vi "Pfeiffer-RVC300.set flow.vi"(0 "i ref in":refnum<vi>, 1 "flow":dbl, 3 "ms timeout (10000)":i32=10000, 5 "error in (no error)":errorcluster) -> (14 "i ref out":refnum<vi>, 17 "timed out":bool, 19 "error out":errorcluster)   [LabVIEW 2014, in "Pfeiffer-RVC300.lvlib"]
doc: "Sets the flow for flow regulation.\n\nLicense Agreement for this software:\n\nCopyright (C)\nMax-Planck-Institut für Kernphysik\nSaupfercheckweg 1\n69117 Heidelberg\nGermany\n\nContact: christopher.borgmann@mpi-hd.mpg.de\n\nThis program is free software: you can redistribute it and/or modify \nit under the terms of the GNU General Public License as published by\nthe Free Software Foundation, either version 3 of the License, or\n(at your option) any later version.\n\nThis program is distributed in the hope that it will be useful,\nbut WITHOUT ANY WARRANTY; without even the implied warranty of\nMERCHANTABILITY or FITNESS FOR A PARTICULAR PURPOSE. See the\nGNU General Public License for more details.\n\nYou should have received a copy of the GNU General Public License\nalong with this program. If not, see <http://www.gnu.org/licenses/>.\n\nMax-Planck-Institut für Kernphysik\nSaupfercheckweg 1, 69117 Heidelberg, Germany\nFor all questions and ideas contact: christopher.borgmann@mpi-hd.mpg.de\nLast update: 08.07.2010"
uses:
  Pfeiffer-RVC300.lvlib
  CSCore/CSApplicationBaseClasses/DeviceBase/DeviceBase.lvlib
  CSlibraries-extern/DimLVEvent/LVDimInterface/LVDimInterface.lvlib
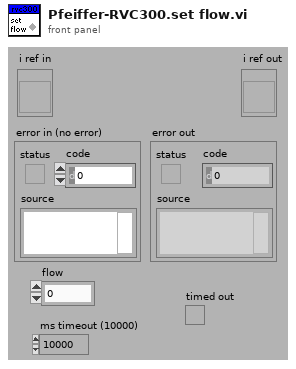
[diagram p1: front panel]
types:
  T1 = typedef "Pfeiffer-RVC300.lvlib/Pfeiffer-RVC300.i attribute.ctl" = cluster{"interfaceInitialized":bool, "VISAResource":refnum<visa-resource-name>, "WaitingTime":u32, "nomValues":T2, "actValues":T2}
  T2 = typedef "Pfeiffer-RVC300.lvlib/Pfeiffer-RVC300.parameters.ctl" = cluster{"regulationMode":T3, "valveType":string, "sensorType":string, "valveState":string, "flow":dbl, "pressure":dbl, "serviceIDs":cluster{"regulationModeID":i32, "valveTypeID":i32, "sensorTypeID":i32, "valveStateID":i32, "flowID":i32, "pressureID":i32}}
  T3 = typedef "Pfeiffer-RVC300.lvlib/Pfeiffer-RVC300.regulation mode.ctl" = enum16{"unknown", "Pressure", "Flow", "Wait"}
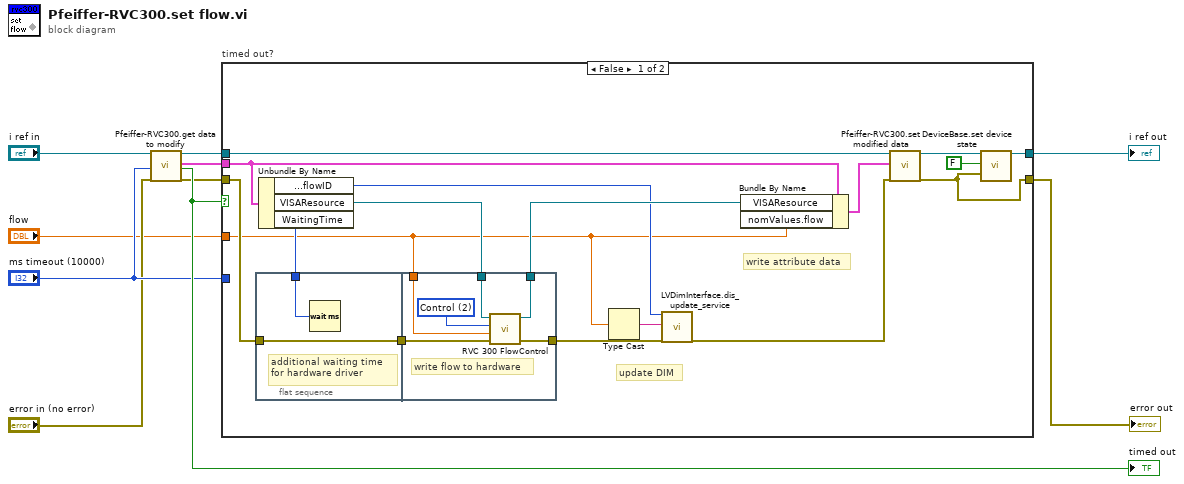
[diagram p0: block diagram]
diagram:
  n1 = call "Pfeiffer-RVC300.get data to modify.vi"("i ref in"="i ref in", "ms timeout (10000)"="ms timeout (10000)", "error in (no error)"="error in (no error)") -> ("i ref out"=w4:refnum<vi>, "i attribute"=w2:T1, "timed out"=w7:bool, "error out"=w3:errorcluster)  [unwired: 13 in]
  "timed out" <- w7
  n2 = case "timed out?" shown="False" w7 {
    tunnel: [w24 w37] -> w9
    tunnel: w4 -> [w27 w37]
    tunnel: [w22 w36] -> w8
    tunnel: w3 -> [w21 w36]
    tunnel: w2 -> [w19 _]
    tunnel: "ms timeout (10000)" -> [_ _]
    tunnel: "flow" -> [w11 _]
    frame False {
      # "write attribute data"
      # "update DIM"
      n3 = flat-sequence {
        tunnel: w21 -> [w29]
        tunnel: [w29] -> w20
        tunnel: w16 -> [w28]
        tunnel: w20 -> [w35]
        tunnel: w17 -> [w32]
        tunnel: [w34] -> w12
        tunnel: [w33] -> w18
        tunnel: w11 -> [w30]
        frame #0 {
          # "additional waiting time \nfor hardware driver"
          n4 = Wait (ms)(milliseconds to wait=w28) -> ()  [unwired: 1 out]
        }
        frame #1 {
          w31 = u16 2 items=["Close", "Open", "Control"] ("Action")
          # "write flow to hardware"
          n5 = call "RVC 300 FlowControl.vi"("error in"=w35, "Flow"=w30, "Action"=w31, "Resource Name"=w32) -> ("error out"=w34:errorcluster, "Resource Name out"=w33:refnum<visa-resource-name>)  [unwired: 5 in, 1 out]
        }
      }
      n6 = Unbundle By Name(w19) -> ("nomValues.serviceIDs.flowID"=w15:i32, "VISAResource"=w17:refnum<visa-resource-name>, "WaitingTime"=w16:u32)
      n7 = Type Cast(x=w11) -> (*(type *) &x=w14:string)  [unwired: 1 in]
      n8 = call "LVDimInterface.dis_update_service.vi"("my_serviceID"=w15, "data"=w14, "error in (no error)"=w12) -> ("error out"=w13:errorcluster)  [unwired: 14 in, 2 out]
      n9 = Bundle By Name(cluster=w19, "VISAResource"=w18, "nomValues.flow"=w11) -> (w26:T1)
      n10 = call "Pfeiffer-RVC300.set modified data.vi"("i ref in"=w27, "i attribute"=w26, "error in (no error)"=w13) -> ("i ref out"=w25:refnum<vi>, "error out"=w22:errorcluster)  [unwired: 15 in]
      n11 = call "DeviceBase.set device state.vi"("i ref in"=w25, "implicit"=FALSE, "device error"=w22) -> ("i ref out"=w24:refnum<vi>)  [unwired: 14 in, 2 out]
    }
    frame True {
    }
  }
  "error out" <- w8
  "i ref out" <- w9
